vi "PiezoJenaNanoBox.vi"() -> ()   [LabVIEW 2011]
uses:
  <vilib>/Instr/_visa.llb/VISA Flush IO Buffer Mask.ctl
panel:
  out "error out":errorcluster
  out "read buffer":string
  out "Return":string
  in  "Ring":u16(ring) items=["stat", "err", "idn", "serno", "cl,0", "cl,1", "hvon,0", "hvon,1", "rst", "ki"]
  out "Waveform Chart":T1(graph)
  in  "send":bool
  in  "CL":bool caption="OL"
  in  "Volt":dbl(slide) scale=0.0..128.0
  in  "soll position":dbl(slide) scale=0.0..120.0
  in  "stop, close com":bool
  in  "VISA resource name":refnum<visa-resource-name>
  # "Kommando Funktion\nidn Geräteidentifikation\nrst Softwarereset\nbreak Unterbrechung der laufenden Ausgabe\nstart Startet Funktionsgenerator oder Arbitrary(Tabellen)-Funktion\nstop Abbruch der laufenden Ausgabe\nstat Status abfragen\nerr Fehlerstatus abfragen\ndef Konfiguration des Gerätes\ndefp Konfiguration der Default-Werte\nhvon Hochspannung schalten\nvolt Sollwert für Piezospannung setzen oder lesen\nmvolt liest den DAC der Ausgangsspannung\npos Position setzen oder lesen\nmpos liest das Messsystem und gibt die aktuelle Position zurück\nsens Sensor abfragen\ncl Driftausgleich ein- oder ausschalten\nki Parameter Driftausgleich\nsin Sinusfunktion initialisieren oder rücklesen\nrect Rechteckfunktion initialisieren oder rücklesen\ntria Dreieckfunktion initialisieren oder rücklesen\ntbres Tabelle rücksetzen\ntbpos Tabellenwertepaar setzen oder rücklesen\ntblo untere Grenze des Ausgabezeigers setzen oder rücklesen\ntbhi obere Grenze des Ausgabezeigers setzen oder rücklesen\ntbptr Ausgabezeiger setzen oder rücklesen\ntbval Tabellenwertepaare mit automatischen Zeigerinkrement setzen oder rücklesen\nresgen Arbitrary-Tabelle und Funktionsgenerator zurücksetzen\nversion ruft die Versionsnummer der Firmware ab\nserno ruft die Seriennummer der nano box USB ab\ns zeigt die Kommandoliste an"
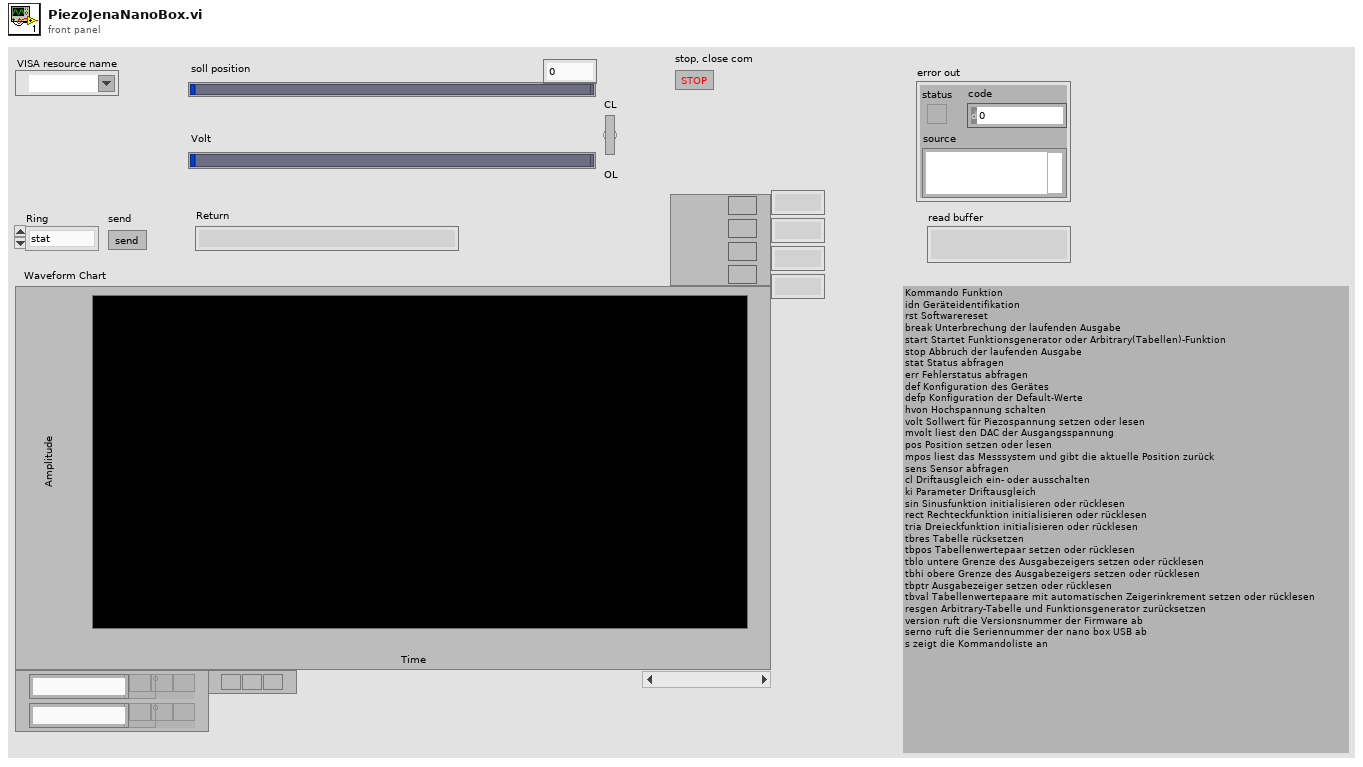
[diagram p1: front panel]
types:
  T1 = cluster{"[0]":dbl, "[1]":dbl, "[2]":dbl, "[3]":dbl}
  T2 = typedef "VISA Flush IO Buffer Mask.ctl" = u16
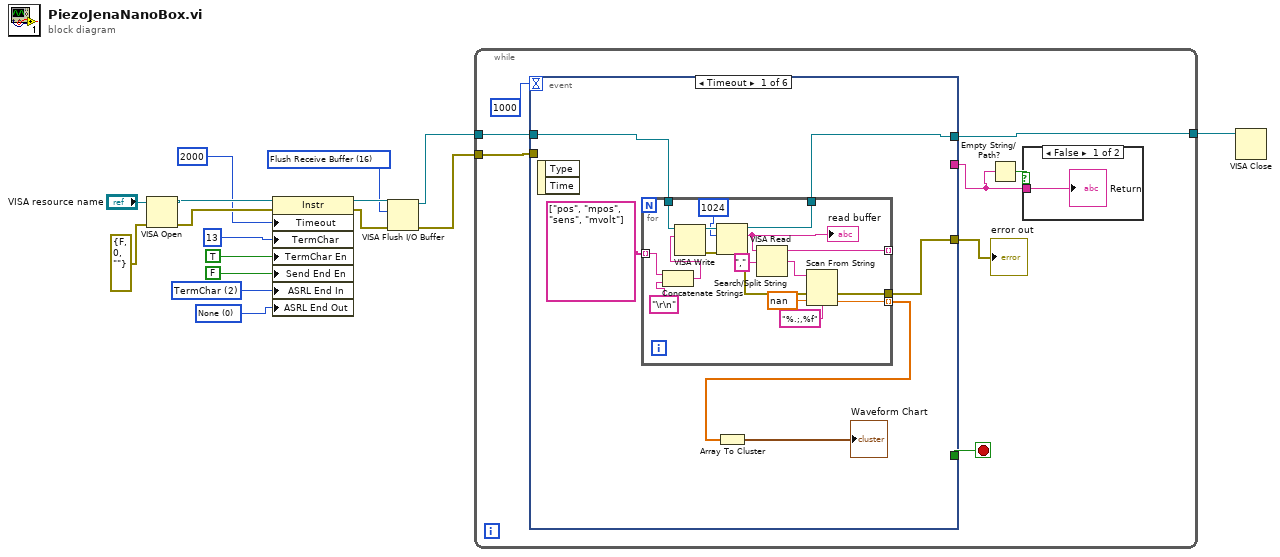
[diagram p0: block diagram]
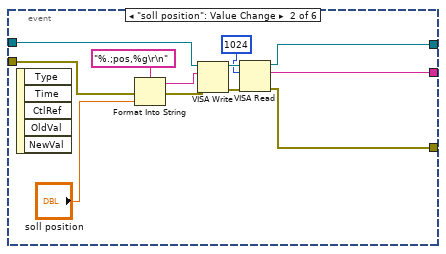
[diagram p3: hidden frame]
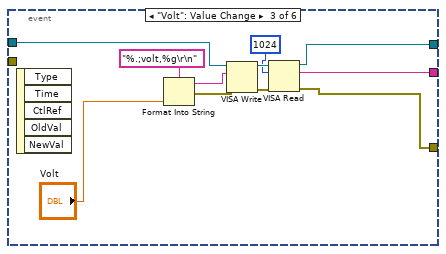
[diagram p4: hidden frame]
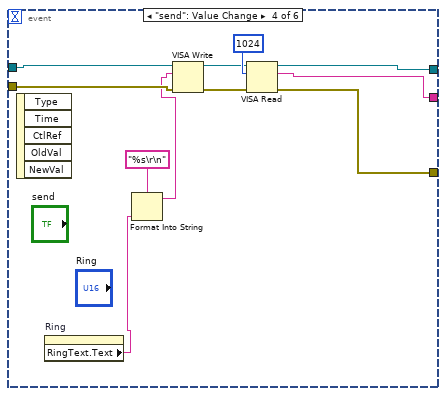
[diagram p5: hidden frame]
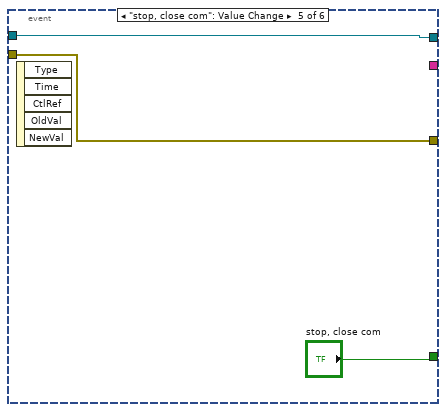
[diagram p6: hidden frame]
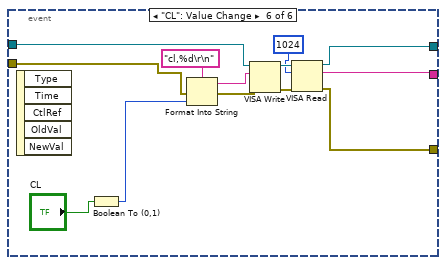
[diagram p7: hidden frame]
diagram:
  w4 = T2 16 items=["Flush Receive Buffer"=16, "Write Transmit Buffer to Device"=32, "Flush Receive Buffer (No I/O)"=64, "Flush Transmit Buffer"=128] ("Mask")
  w8 = u16 0 items=["None", "Last Bit", "TermChar", "Break"] ("Serial Settings:End Mode for Writes")
  w9 = u16 2 items=["None", "Last Bit", "TermChar"] ("Serial Settings:End Mode for Reads")
  n1 = VISA Open(error in (no error)=errorcluster {"status"=FALSE, "code"=0, "source"=""}, VISA resource name="VISA resource name") -> (VISA resource name=w10:refnum<visa-resource-name>, error out=w11:errorcluster)  [unwired: 3 in]
  n2 = property class="Instr"(reference=w10, error in=w11, "Timeout"=u32 2000 ("timeout [ms] (10000)"), "TermChar"=u8 13 ("Message Based Settings:Termination Character"), "TermChar En"=TRUE, "Send End En"=FALSE, "ASRL End In"=w9, "ASRL End Out"=w8) -> (reference out=w6:refnum<visa-resource-name>, error out=w5:errorcluster)
  n3 = VISA Flush I/O Buffer(VISA resource name=w6, mask (16)=w4, error in (no error)=w5) -> (VISA resource name out=w3:refnum<visa-resource-name>, error out=w2:errorcluster)
  n4 = while {
    tunnel: w3 -> [w23]
    tunnel: w2 -> [w22]
    tunnel: [w20] -> w1
    stop <- w24 stop-if-true
    n5 = event shown="[0] Timeout" {
      selector: _ -> [_ _ _ _ _ _]
      dyn-events: _ -> [_ _ _ _ _ _]
      timeout: 1000 -> [_ _ _ _ _ _]
      tunnel: [_ _ _ _ "stop, close com" _] -> w24
      tunnel: w23 -> [w30 w57 w65 w80 w84 w92]
      tunnel: w22 -> [_ w52 _ w79 w83 w88]
      tunnel: [w29 w56 w63 w74 w84 w91] -> w20
      tunnel: [w26 w50 w62 w73 w83 w87] -> w19
      tunnel: [_ w49 w61 w72 _ w86] -> w18
      event Timeout {
        n6 = event-data() -> ()  [unwired: 1 in, 2 out]
        n7 = for {
          tunnel: string[] ["pos", "mpos", "sens", "mvolt"] -> [w48] mode=indexing
          tunnel: w30 -> [w46]
          tunnel: [w41] -> w29
          tunnel: [w39] -> w28 mode=indexing
          tunnel: [w37] -> _ mode=indexing
          tunnel: [w34] -> w26
          n8 = Concatenate Strings(w48, "\r\n" ("format string")) -> (w45:string)
          n9 = VISA Write(VISA resource name=w46, write buffer=w45) -> (VISA resource name out=w44:refnum<visa-resource-name>, error out=w42:errorcluster)  [unwired: 1 in, 1 out]
          n10 = VISA Read(VISA resource name=w44, byte count=u32 1024, error in (no error)=w42) -> (VISA resource name out=w41:refnum<visa-resource-name>, read buffer=w33:string, error out=w35:errorcluster)  [unwired: 1 out]
          "read buffer" <- w33
          n11 = Search/Split String(string=w33, search string/char (-)=",") -> (substring before match=w37:string, match + rest of string=w36:string)  [unwired: 1 in, 1 out]
          n12 = Scan From String(format string="%.;,%f", input string=w36, error in=w35, default 1=nan ("default value 1")) -> (error out=w34:errorcluster, output 1=w39:dbl)  [unwired: 1 in, 2 out]
        }
        n13 = Array To Cluster(array=w28) -> (cluster=→"Waveform Chart":T1)
      }
      event "soll position": Value Change {
        n14 = event-data() -> ()  [unwired: 1 in, 5 out]
        n15 = Format Into String(format string="%.;pos,%g\r\n", error in=w52, "soll position") -> (resulting string=w53:string, error out=w51:errorcluster)  [unwired: 1 in]
        n16 = VISA Write(VISA resource name=w57, write buffer=w53, error in (no error)=w51) -> (VISA resource name out=w60:refnum<visa-resource-name>, error out=w58:errorcluster)  [unwired: 1 out]
        n17 = VISA Read(VISA resource name=w60, byte count=u32 1024, error in (no error)=w58) -> (VISA resource name out=w56:refnum<visa-resource-name>, read buffer=w49:string, error out=w50:errorcluster)  [unwired: 1 out]
      }
      event "Volt": Value Change {
        n18 = event-data() -> ()  [unwired: 1 in, 5 out]
        n19 = Format Into String(format string="%.;volt,%g\r\n", "Volt") -> (resulting string=w67:string, error out=w66:errorcluster)  [unwired: 2 in]
        n20 = VISA Write(VISA resource name=w65, write buffer=w67, error in (no error)=w66) -> (VISA resource name out=w71:refnum<visa-resource-name>, error out=w69:errorcluster)  [unwired: 1 out]
        n21 = VISA Read(VISA resource name=w71, byte count=u32 1024, error in (no error)=w69) -> (VISA resource name out=w63:refnum<visa-resource-name>, read buffer=w61:string, error out=w62:errorcluster)  [unwired: 1 out]
      }
      event "send": Value Change {
        n22 = event-data() -> ()  [unwired: 1 in, 5 out]
        n23 = property on="Ring" class="Ring (strict)"() -> ("RingText.Text"=w81:string)  [unwired: 2 in, 2 out]
        n24 = Format Into String(format string="%s\r\n", w81) -> (resulting string=w78:string)  [unwired: 2 in, 1 out]
        n25 = VISA Write(VISA resource name=w80, write buffer=w78, error in (no error)=w79) -> (VISA resource name out=w76:refnum<visa-resource-name>, error out=w75:errorcluster)  [unwired: 1 out]
        n26 = VISA Read(VISA resource name=w76, byte count=u32 1024, error in (no error)=w75) -> (VISA resource name out=w74:refnum<visa-resource-name>, read buffer=w72:string, error out=w73:errorcluster)  [unwired: 1 out]
      }
      event "stop, close com": Value Change {
        n27 = event-data() -> ()  [unwired: 1 in, 5 out]
      }
      event "CL": Value Change {
        n28 = event-data() -> ()  [unwired: 1 in, 5 out]
        n29 = Boolean To (0,1)(Boolean="CL") -> (0, 1=w89:i16)
        n30 = Format Into String(format string="cl,%d\r\n", error in=w88, w89) -> (resulting string=w94:string, error out=w93:errorcluster)  [unwired: 1 in]
        n31 = VISA Write(VISA resource name=w92, write buffer=w94, error in (no error)=w93) -> (VISA resource name out=w98:refnum<visa-resource-name>, error out=w96:errorcluster)  [unwired: 1 out]
        n32 = VISA Read(VISA resource name=w98, byte count=u32 1024, error in (no error)=w96) -> (VISA resource name out=w91:refnum<visa-resource-name>, read buffer=w86:string, error out=w87:errorcluster)  [unwired: 1 out]
      }
    }
    "error out" <- w19
    n33 = Empty String/Path?(string/path=w18) -> (empty?=w17:bool)
    n34 = case shown="False" w17 {
      tunnel: w18 -> [w25 _]
      frame False {
        "Return" <- w25
      }
      frame True {
      }
    }
  }
  n35 = VISA Close(VISA resource name=w1) -> ()  [unwired: 1 in, 1 out]
